vi "Save Library for Previous.vi"(6 "Save Version":string, 7 "Library Path":path, 8 "error in":errorcluster, 11 "Library Icon Data in":refnum<class "Library Icon Data.lvclass">) -> (0 "error out":errorcluster, 3 "Library Icon Data out":refnum<class "Library Icon Data.lvclass">)   [LabVIEW 2020, in "Library Icon Data.lvclass"]
doc: "Saves the library in the specified LabVIEW version."
uses:
  Library Icon Data.lvclass
  Library Icon Data.lvclass/Library Icon Data.ctl
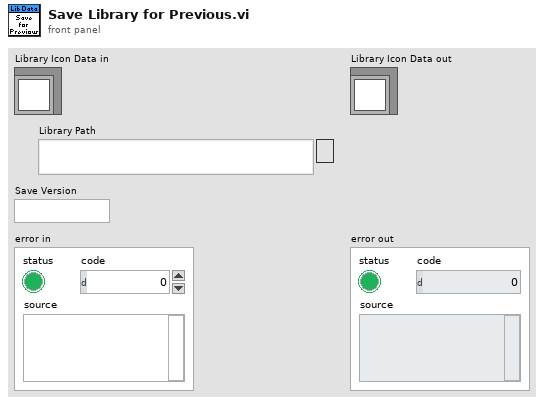
[diagram p1: front panel]
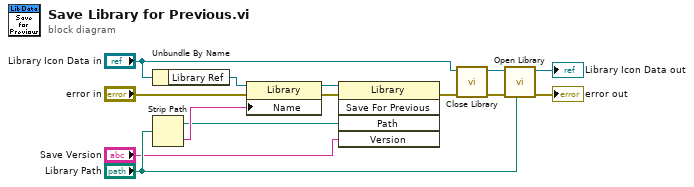
[diagram p0: block diagram]
diagram:
  n1 = Unbundle By Name("Library Icon Data in") -> ("Library Ref"=w8:refnum<vi>)
  n2 = Strip Path(path="Library Path") -> (stripped path=w6:path, name=w9:string)
  n3 = property class="Library"(reference=w8, error in="error in", "Name"=w9) -> (reference out=w7:refnum<vi>, error out=w13:errorcluster)
  n4 = invoke class="Library" method="Save For Previous"(reference=w7, error in=w13, "Path"=w6, "Version"="Save Version") -> (error out=w12:errorcluster)  [unwired: 1 in, 4 out]
  n5 = call "Close Library.vi"("error in"=w12, "Library Icon Data in"="Library Icon Data in") -> ("error out"=w11:errorcluster, "Library Icon Data out"=w5:refnum<class "Library Icon Data.lvclass">)  [unwired: 8 in]
  n6 = call "Open Library.vi"("Library Path"="Library Path", "error in"=w11, "Library Icon Data in"=w5) -> ("error out"=→"error out":errorcluster, "Library Icon Data out"=→"Library Icon Data out":refnum<class "Library Icon Data.lvclass">)  [unwired: 7 in]
